vi "SVL Get Spectrum Subset (1 Ch).vi"(0 "spectrum":cluster{"x0":dbl, "dx":dbl, "magnitude":dbl[]} {"magnitude" format="%.2f"; "dx" format="%.2f"; "x0" format="%.2f"}, 2 "range":cluster{"start":dbl, "stop":dbl}={"start"=-1.0, "stop"=-1.0} {"stop" format="%.2f"; "start" format="%.2f"}, 4 "spectrum info":T1={"channel name"="", "description"="", "x-axis units"=0, "spectral info"={"spectrum type"=enum."Power [Magnitude^2]", "linear/dB"=enum."linear", "window"=0, "window size"=0, "FFT size"=0}, "engineering units"=0, "custom label"="", "dB reference [EU]"=0.0, "peak units"=enum."rms", "weighting filter"=0, "spectral density?"=FALSE, "unit label"="", "spectrum skewed?"=FALSE, "complimentary spectrum units"=enum."none"} {"x-axis units" items=["Time (s)"=0, "Frequency-CB (Hz)"=1, "Frequency-CPB (Hz)"=1248, "Frequency-Arbitrary (Hz)"=2357, "Quefrency (s)"=2, "Revolutions (rev)"=3, "Order"=4, "Speed (RPM)"=11, "Speed (rad/s)"=21, "Index"=65535]; "weighting filter" items=["Linear", "A-weighting", "B-weighting", "C-weighting", "ITU-R 468-4", "Dolby", "CCITT", "C-message", "Wb", "Wc", "Wd", "We", "Wf", "Wh", "Wj", "Wk", "Wm", "AES17 20 kHz lowpass", "AES17 40 kHz lowpass", "AES17 20 kHz highpass", "AES17 40 kHz highpass"]; "dB reference [EU]" format="%.2f"; "engineering units" items=["custom..."=0, "V"=1, "A"=21, "C"=30, "pC"=31, "s"=32, "-"=29, "Pa"=2, "N"=20, "g"=3, "m/s^2"=4, "m/s"=5, "m"=6, "mm/s"=12, "mm"=13, "micron/s"=14, "micron"=15, "in/s^2"=7, "in/s"=8, "in"=9, "mil/s"=10, "mil"=11, "rad/s^2"=16, "rad/s"=17, "rad"=18, "deg/s^2"=26, "deg/s"=27, "deg"=28, "RPM"=22, "cycle/s^2"=23, "Hz"=24, "cycle"=25, "strain"=19]; "spectral info"."window" items=["None "=0, "Hanning"=1, "Hamming"=2, "Blackman-Harris"=3, "Exact Blackman"=4, "Blackman"=5, "Flat Top"=6, "4 Term B-Harris "=7, "7 Term B-Harris"=8, "Low Sidelobe"=9, "Force - Exponential"=10, "Gaussian"=62]}, 5 "error in (no error)":errorcluster) -> (14 "spectrum subset":cluster{"x0":dbl, "dx":dbl, "magnitude":dbl[]} {"magnitude" format="%.2f"; "dx" format="%.2f"; "x0" format="%.2f"}, 15 "unit label":string, 16 "actual range":cluster{"start":dbl, "stop":dbl}={"start"=-1.0, "stop"=-1.0} {"stop" format="%.2f"; "start" format="%.2f"}, 17 "range label":string, 18 "dup spectrum info":T1={"channel name"="", "description"="", "x-axis units"=0, "spectral info"={"spectrum type"=enum."Power [Magnitude^2]", "linear/dB"=enum."linear", "window"=0, "window size"=0, "FFT size"=0}, "engineering units"=0, "custom label"="", "dB reference [EU]"=0.0, "peak units"=enum."rms", "weighting filter"=0, "spectral density?"=FALSE, "unit label"="", "spectrum skewed?"=FALSE, "complimentary spectrum units"=enum."none"} {"x-axis units" items=["Time (s)"=0, "Frequency-CB (Hz)"=1, "Frequency-CPB (Hz)"=1248, "Frequency-Arbitrary (Hz)"=2357, "Quefrency (s)"=2, "Revolutions (rev)"=3, "Order"=4, "Speed (RPM)"=11, "Speed (rad/s)"=21, "Index"=65535]; "weighting filter" items=["Linear", "A-weighting", "B-weighting", "C-weighting", "ITU-R 468-4", "Dolby", "CCITT", "C-message", "Wb", "Wc", "Wd", "We", "Wf", "Wh", "Wj", "Wk", "Wm", "AES17 20 kHz lowpass", "AES17 40 kHz lowpass", "AES17 20 kHz highpass", "AES17 40 kHz highpass"]; "dB reference [EU]" format="%.2f"; "engineering units" items=["custom..."=0, "V"=1, "A"=21, "C"=30, "pC"=31, "s"=32, "-"=29, "Pa"=2, "N"=20, "g"=3, "m/s^2"=4, "m/s"=5, "m"=6, "mm/s"=12, "mm"=13, "micron/s"=14, "micron"=15, "in/s^2"=7, "in/s"=8, "in"=9, "mil/s"=10, "mil"=11, "rad/s^2"=16, "rad/s"=17, "rad"=18, "deg/s^2"=26, "deg/s"=27, "deg"=28, "RPM"=22, "cycle/s^2"=23, "Hz"=24, "cycle"=25, "strain"=19]; "spectral info"."window" items=["None "=0, "Hanning"=1, "Hamming"=2, "Blackman-Harris"=3, "Exact Blackman"=4, "Blackman"=5, "Flat Top"=6, "4 Term B-Harris "=7, "7 Term B-Harris"=8, "Low Sidelobe"=9, "Force - Exponential"=10, "Gaussian"=62]}, 19 "error out":errorcluster)   [LabVIEW 2017]
doc: "Extracts the subset of the spectrum specified by <B>range</B>. <B>x0</B> is updated to reflect the new start frequency, <B>dx</B> is the same as in the input spectrum, and the spectrum array is shortened so the last element corresponds with the stop value specified in the <B>range</B>. Use this VI for operations such as limiting subsequent spectrum operations to the region of interest or removing the part of the spectrum outside the alias-free bandwidth, as well as others. You can use this polymorphic VI to take a subset of a single spectrum, N spectra, a single complex spectrum, or N complex spectra. The data type you wire to the <B>phase spectrum</B> input determines the polymorphic instance to use."
uses:
  <vilib>/addons/_NISVFA/_Shared subVIs/Controls/svc_Spectrum Info.ctl
  <vilib>/addons/_NISVFA/_Shared subVIs/Controls/svc_X-Axis Units.ctl
  <vilib>/addons/_NISVFA/_Shared subVIs/Controls/svc_Spectrum Type.ctl
  <vilib>/addons/_NISVFA/_Shared subVIs/Controls/svc_Engineering Units Text Ring.ctl
  <vilib>/addons/_NISVFA/_Shared subVIs/Controls/svc_Weighting Filter Text Ring.ctl
  <vilib>/addons/_NISVFA/_Shared subVIs/Controls/svc_Complimentary Spectrum Units.ctl
  <vilib>/addons/_NISVFA/_Shared subVIs/Common/svc_Get Weighting Enum and Labels.vi
  <vilib>/addons/_NISVFA/_Shared subVIs/Common/svc_Unit Label Lexical Class.vi
  <vilib>/addons/_NISVFA/_Shared subVIs/Common/svc_Engineering Units to Unit Label.vi
  <vilib>/addons/_NISVFA/_Shared subVIs/Common/svc_Format Value (DBL).vi
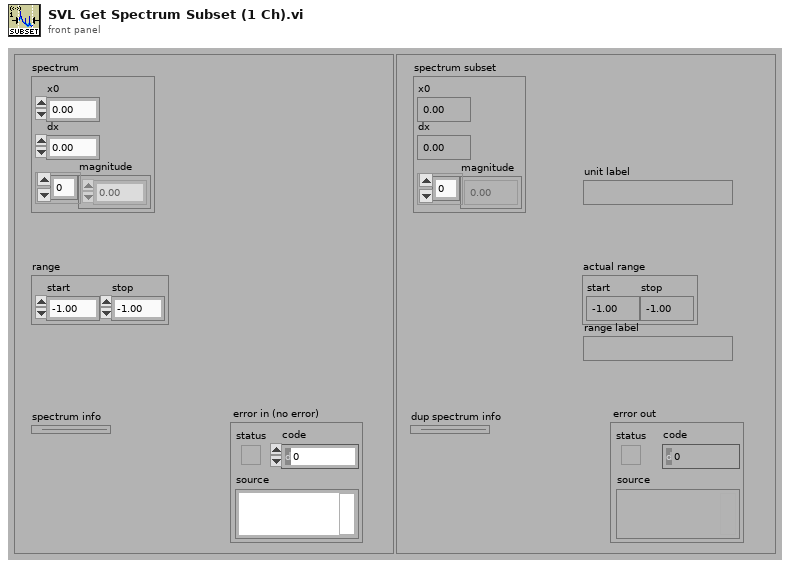
[diagram p1: front panel]
types:
  T1 = typedef "svc_Spectrum Info.ctl" = cluster{"channel name":string, "description":string, "x-axis units":T2, "spectral info":cluster{"spectrum type":T3, "linear/dB":enum16{"linear", "dB"}, "window":u16, "window size":i32, "FFT size":i32}, "engineering units":T4, "custom label":string, "dB reference [EU]":dbl, "peak units":enum16{"rms", "peak", "peak-peak"}, "weighting filter":T5, "spectral density?":bool, "unit label":string, "spectrum skewed?":bool, "complimentary spectrum units":T6}
  T2 = typedef "svc_X-Axis Units.ctl" = u16
  T3 = typedef "svc_Spectrum Type.ctl" = enum16{"FFT Spectrum [complex]", "Amplitude [Magnitude]", "Power [Magnitude^2]", "Cross Spectrum [complex]", "Frequency Response [Complex]"}
  T4 = typedef "svc_Engineering Units Text Ring.ctl" = u16
  T5 = typedef "svc_Weighting Filter Text Ring.ctl" = u16
  T6 = typedef "svc_Complimentary Spectrum Units.ctl" = enum16{"none", "radians", "degrees", "cycles", "imaginary"}
  T7 = cluster{"start frequency":dbl, "stop frequency":dbl}
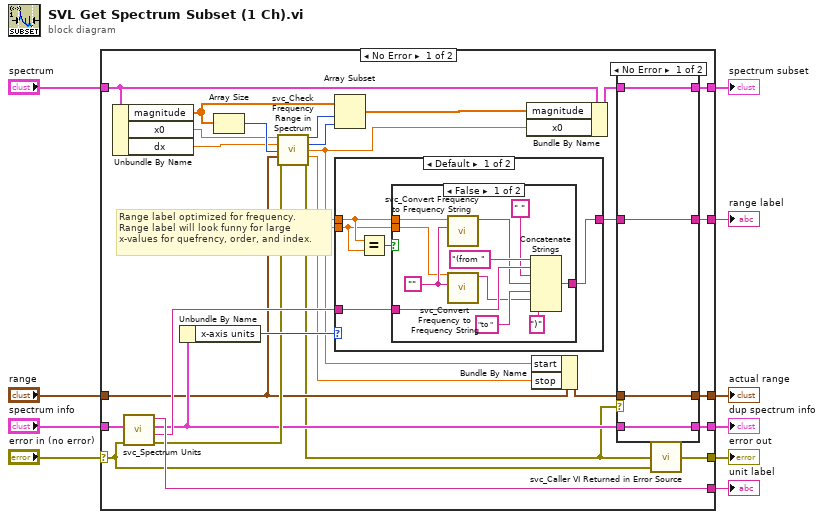
[diagram p0: block diagram]
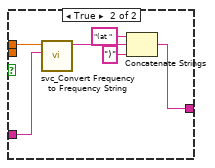
[diagram p2: hidden frame]
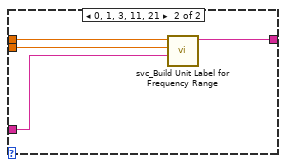
[diagram p3: hidden frame]
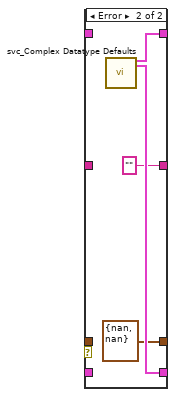
[diagram p4: hidden frame]
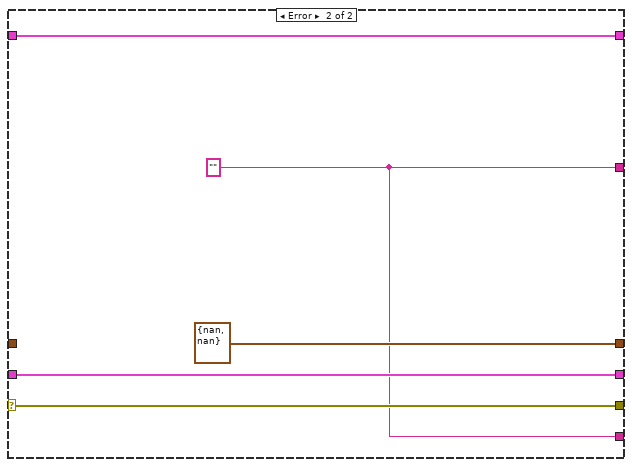
[diagram p5: hidden frame]
diagram:
  n1 = case shown="No Error" "error in (no error)" {
    selector: "error in (no error)" -> [w11 w75]
    tunnel: [w25 w76] -> w10
    tunnel: "range" -> [w15 _]
    tunnel: "spectrum" -> [w30 w76]
    tunnel: [w24 w72] -> w6
    tunnel: [w22 w74] -> w3
    tunnel: "spectrum info" -> [w18 w74]
    tunnel: [w23 T7 {"start frequency"=nan, "stop frequency"=nan} ("frequency range")] -> w2
    tunnel: [w12 w75] -> w9
    tunnel: [w26 w72] -> w1
    frame No Error {
      # "Range label optimized for frequency.\nRange label will look funny for large \nx-values for quefrency, order, and index."
      n2 = Unbundle By Name(w30) -> ("magnitude"=w31:dbl[], "x0"=w33:dbl, "dx"=w32:dbl)
      n3 = call <vilib>:"svc_Spectrum Units.vi"("error in (no error)"=w11, "spectrum info in"=w18) -> ("error out"=w19:errorcluster, "x-axis unit label"=w20:string, "spectrum info out"=w17:T1, "unit label"=w26:string)  [unwired: 2 in]
      n4 = Unbundle By Name(w17) -> ("x-axis units"=w21:T2)
      n5 = Array Size(array=w31) -> (size(s)=w34:i32)
      n6 = call <vilib>:"svc_Check Frequency Range in Spectrum.vi"("f0"=w33, "df"=w32, "spectrum length"=w34, "frequency range"=w15, "error in (no error)"=w19) -> ("start index"=w36:i32, "band length"=w37:i32, "f0"=w16:dbl, "fmax"=w14:dbl, "error out"=w13:errorcluster)  [unwired: 6 in]
      n7 = Array Subset(array=w31, index=w36, length=w37) -> (w35:dbl[])
      n8 = case shown="Default" w21 {
        tunnel: w14 -> [w39 w63]
        tunnel: w16 -> [w40 w62]
        tunnel: [w41 w61] -> w28
        tunnel: w20 -> [w42 w60]
        frame Default {
          n9 = Equal?(x=w40, y=w39) -> (x = y?=w38:bool)
          n10 = case shown="False" w38 {
            tunnel: w42 -> [w51 w58]
            tunnel: [w47 w54] -> w41
            tunnel: w40 -> [w46 w59]
            tunnel: w39 -> [w45 _]
            frame False {
              w53 = "" ("Empty String Constant")
              n11 = call <vilib>:"svc_Convert Frequency to Frequency String.vi"("x-axis unit label"=w53, "frequency [Hz]"=w46) -> ("frequency string"=w50:string)  [unwired: 9 in]
              n12 = call <vilib>:"svc_Convert Frequency to Frequency String.vi"("x-axis unit label"=w53, "frequency [Hz]"=w45) -> ("frequency string"=w44:string)  [unwired: 9 in]
              n13 = Concatenate Strings("(from ", w51, " ", w50, "to ", w44, ")") -> (w47:string)
            }
            frame True {
              n14 = call <vilib>:"svc_Convert Frequency to Frequency String.vi"("x-axis unit label"=w58, "frequency [Hz]"=w59) -> ("frequency string"=w56:string)  [unwired: 9 in]
              n15 = Concatenate Strings("(at " ("string"), w56, ")" ("string")) -> (w54:string)
            }
          }
        }
        frame 0, 1, 3, 11, 21 {
          n16 = call <vilib>:"svc_Build Unit Label for Frequency Range.vi"("x-axis unit label"=w60, "fmax"=w63, "f0"=w62) -> ("frequency range string"=w61:string)  [unwired: 8 in]
        }
      }
      n17 = Bundle By Name(cluster=w30, "magnitude"=w35, "x0"=w16) -> (w27:cluster{"x0":dbl, "dx":dbl, "magnitude":dbl[]})
      n18 = Bundle By Name(cluster=w15, "start"=w16, "stop"=w14) -> (w29:cluster{"start":dbl, "stop":dbl})
      n19 = case shown="No Error" w13 {
        tunnel: w29 -> [w65 _]
        tunnel: w28 -> [w66 _]
        tunnel: w27 -> [w67 _]
        tunnel: [w67 w71] -> w25
        tunnel: [w66 "" ("frequency range string")] -> w24
        tunnel: [w65 T7 {"start frequency"=nan, "stop frequency"=nan} ("frequency range")] -> w23
        tunnel: w17 -> [w64 _]
        tunnel: [w64 w70] -> w22
        frame No Error {
        }
        frame Error {
          n20 = call <vilib>:"svc_Complex Datatype Defaults.vi"() -> ("empty spectrum"=w71:cluster{"f0":dbl, "df":dbl, "magnitude":dbl[]}, "dead spectrum info"=w70:T1)  [unwired: 11 in, 7 out]
        }
      }
      n21 = call <vilib>:"svc_Caller VI Returned in Error Source.vi"("warning input to caller"=w11, "error in (no error)"=w13) -> ("error out"=w12:errorcluster)  [unwired: 3 in]
    }
    frame Error {
      w72 = "" ("frequency range string")
    }
  }
  "error out" <- w9
  "spectrum subset" <- w10
  "dup spectrum info" <- w3
  "range label" <- w6
  "actual range" <- w2
  "unit label" <- w1
